vi "Concat _String Improovd Sub.vi"(8 "vochtigheid":string[](array[string]), 9 "temp":string[](array[string]), 11 "timestamp":string) -> (1 "concat out":string)   [LabVIEW 2013]
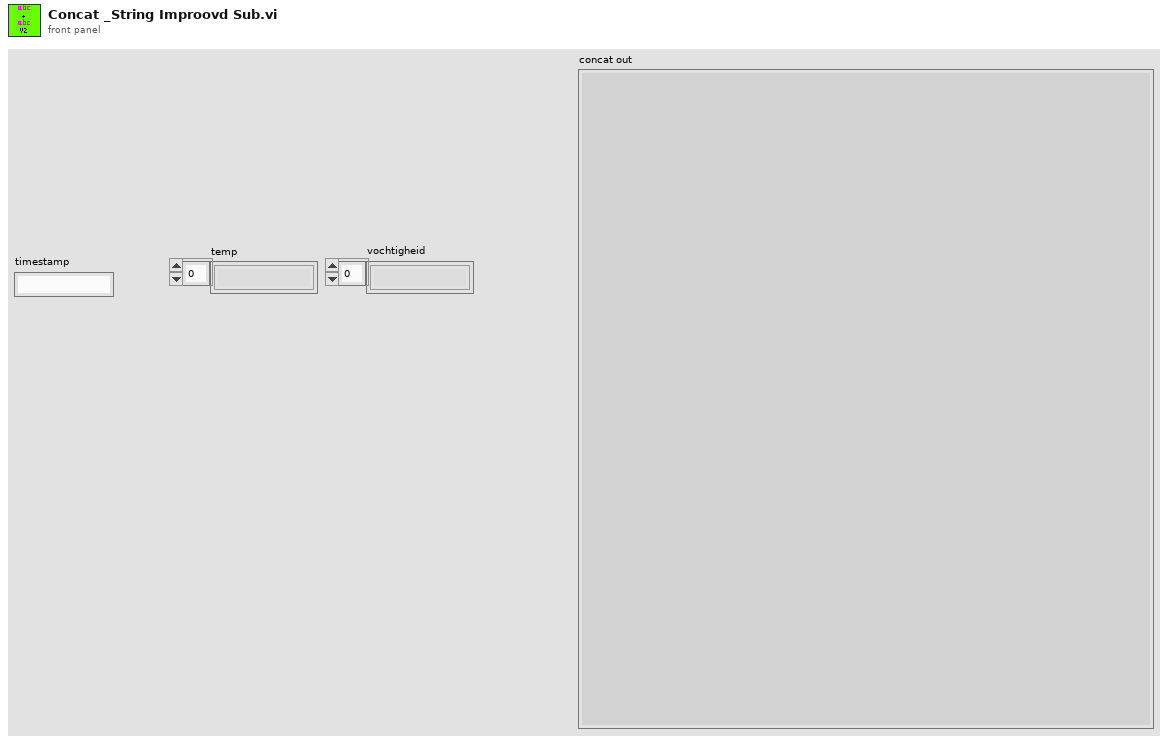
[diagram p1: front panel]
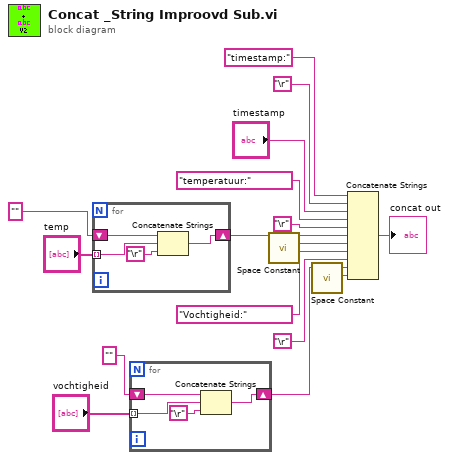
[diagram p0: block diagram]
diagram:
  n1 = for {
    shift-right: [w19] -> w6
    shift-left: "" ("String") -> [w20]
    tunnel: "temp" -> [w18] mode=indexing
    n2 = Concatenate Strings(w20, w18, "\r") -> (w19:string)
  }
  n3 = for {
    shift-right: [w23] -> w2
    shift-left: "" ("String") -> [w24]
    tunnel: "vochtigheid" -> [w22] mode=indexing
    n4 = Concatenate Strings(w24, w22, "\r") -> (w23:string)
  }
  n5 = call <vilib>:"Space Constant.vi"() -> ("String"=w5:string)
  n6 = call <vilib>:"Space Constant.vi"() -> ("String"=w1:string)
  n7 = Concatenate Strings("timestamp:" ("string"), "\r", "timestamp", "temperatuur:" ("string"), "\r", w6, w5, "Vochtigheid:" ("string"), "\r", w2, w1) -> (→"concat out":string)
